vi "ButtonSelectedEnumToBool.vi"(11 "ButtonSelected":enum16{"PID", "Low", "High"}(ring)) -> (1 "PID":bool, 2 "Low":bool, 3 "High":bool)   [LabVIEW 2019, in "XAOMsetting.xctl"]
uses:
  XAOMsetting.xctl
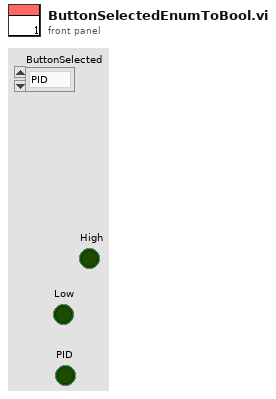
[diagram p1: front panel]
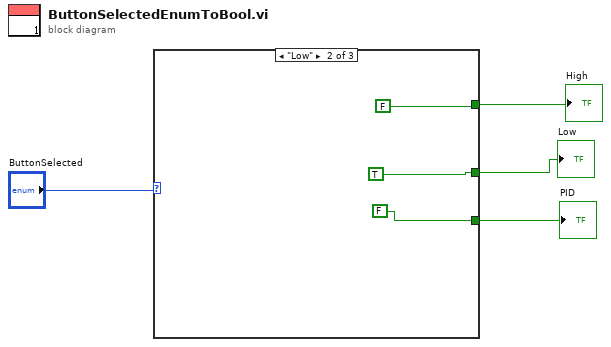
[diagram p0: block diagram]
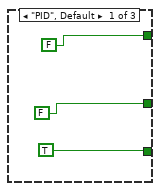
[diagram p2: hidden frame]
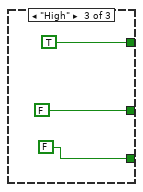
[diagram p3: hidden frame]
diagram:
  n1 = case shown="\"Low\"" "ButtonSelected" {
    tunnel: [FALSE ("High") FALSE ("High") TRUE ("High")] -> w3
    tunnel: [FALSE ("High") TRUE ("High") FALSE ("High")] -> w2
    tunnel: [TRUE ("High") FALSE ("High") FALSE ("High")] -> w1
    frame "PID", Default {
    }
    frame "Low" {
    }
    frame "High" {
    }
  }
  "High" <- w3
  "Low" <- w2
  "PID" <- w1
